vi "Read Config Settings.vi"(8 "error in (no error)":errorcluster, 10 "ConfigFile":path, 11 "Config in":refnum<class "Config.lvclass">) -> (0 "error out":errorcluster, 1 "Config Settings":T1={"Application Settings"={"Simulation"=FALSE}, "Main Settings"={"Simulation"=FALSE, "Signal scaling"=[], "ESR scaling"=[], "num readings to average"=[], "ESR alarm threshhold (%)"=[], "UseDummyVrms"=FALSE, "Dummy Vrms"=0.0, "Inverter Database File"=path "", "default Inverter (name)"=[]}, "DAQ Settings"={"Simulation"=FALSE, "Initial ErrReporting setting"=0, "Initial Measurement settings"={"Data Rate 9775"=3.0, "Data Rate 9215"=1200000.0, "Samples RMS 9215"=480000, "Samples RMS 9775"=3}, "Acquisition mode"=enum."3phase", "DemoMode"=FALSE, "RIO Device"=""}, "LogEngine Settings"={"Simulation"=FALSE, "TDMS_FolderPath"="", "CSV_FolderPath"="", "TDMS_FileName_Prefix"="", "CSV_FileName_Prefix"="", "TDMS_LogDuration(s)"=0.0, "CSV_LogDuration(s)"=0.0}} {"Main Settings"."Dummy Vrms" format="%.2g"; "DAQ Settings"."Initial ErrReporting setting" items=["DONTPRINT", "PRINTWARNINGS", "PRINTFATAL", "PRINTALL"]}, 2 "ConfigFile out":path, 3 "Config out":refnum<class "Config.lvclass">, 4 "default file created":bool)   [LabVIEW 2019, in "Config.lvclass"]
doc: "Developed by Kevin Thompson\nkevin@thompsonengineering.net\n\nCopyright 2018-2020\nThompson Engineering, LLC"
uses:
  Config.lvclass
  DataTypes/Config Settings.ctl
  Application/DataTypes/Settings--cluster.ctl
  Main/DataTypes/Settings--cluster.ctl
  Main/support/Data Algorithms/subvis/DataTypes/Gain control.ctl
  Main/support/Data Algorithms/subvis/DataTypes/ESR scaling--cluster.ctl
  DAQ_Engine/DataTypes/Settings--cluster.ctl
  Common/DataTypes/Measurement Config--cluster.ctl
  Common/DataTypes/Acquisition Mode--cluster.ctl
  Log_Engine/DataTypes/Settings--cluster.ctl
  Config.lvclass/Config.ctl
  Accessors/Set Application Settings.vi
  Accessors/Set Main Settings.vi
  Accessors/Set LogEngine Settings.vi
  <userlib>/_OpenG.lib/file/file.llb/File Exists - Scalar__ogtk.vi
  Accessors/Set DAQ Settings.vi
  Application/Application.lvclass
  DAQ_Engine/DAQ_Engine.lvclass
  Log_Engine/Log_Engine.lvclass
  Main/Main.lvclass
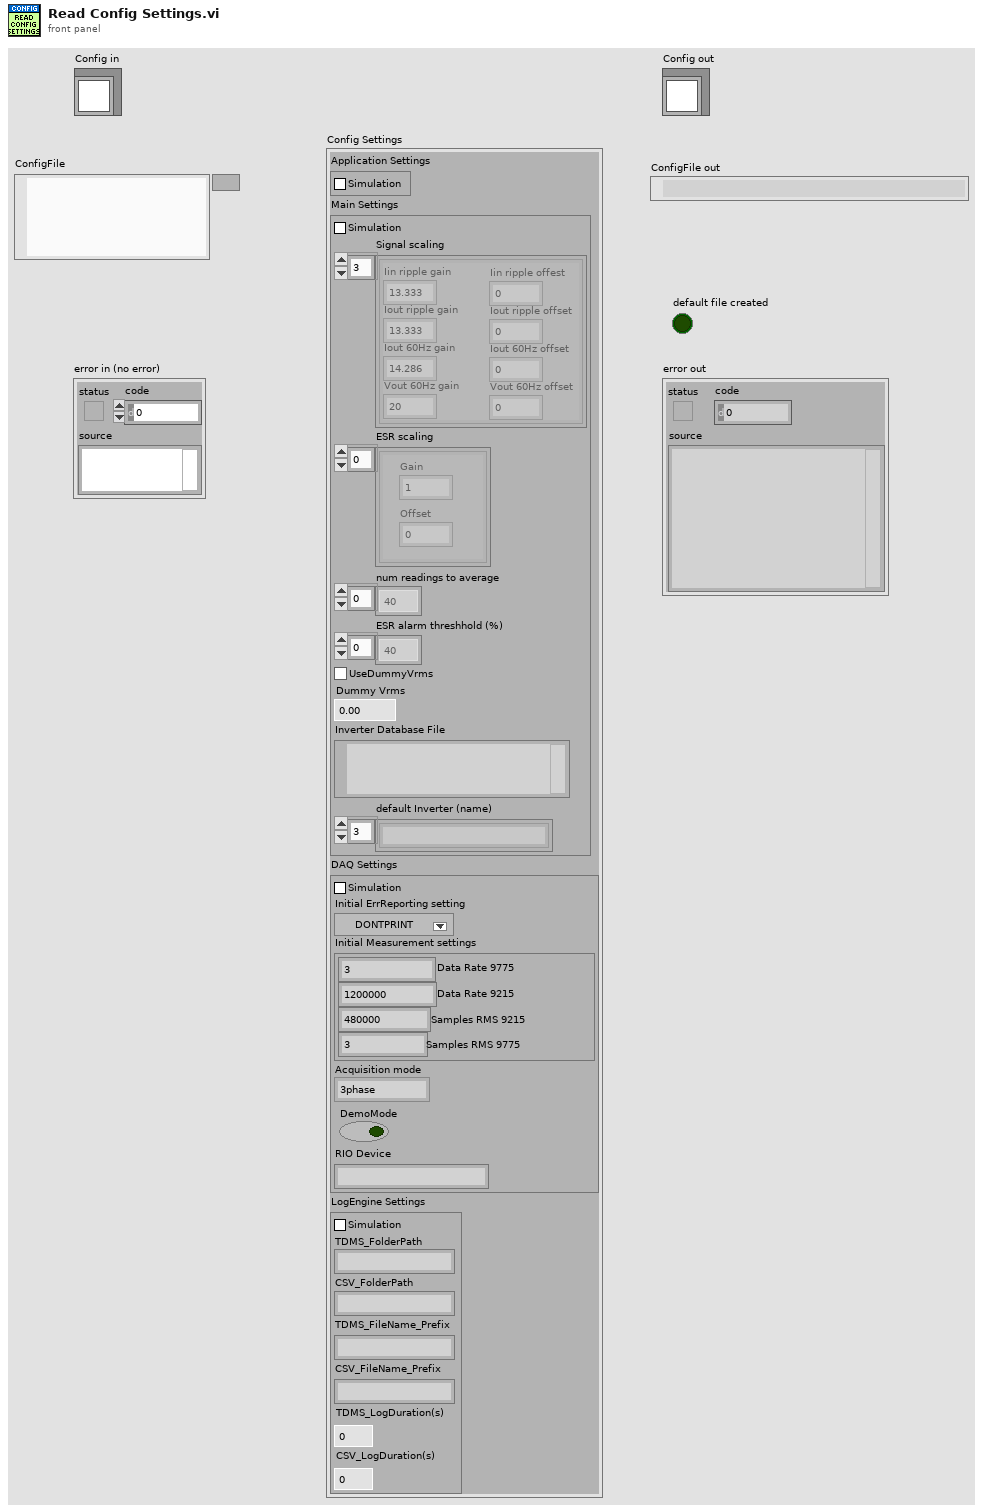
[diagram p1: front panel]
types:
  T1 = typedef "Config.lvclass/Config Settings.ctl" = cluster{"Application Settings":T2, "Main Settings":T3, "DAQ Settings":T6, "LogEngine Settings":T9}
  T2 = typedef "Application.lvclass/Settings--cluster.ctl" = cluster{"Simulation":bool}
  T3 = typedef "Main.lvclass/Settings--cluster.ctl" = cluster{"Simulation":bool, "Signal scaling":T4[], "ESR scaling":T5[], "num readings to average":i32[], "ESR alarm threshhold (%)":i32[], "UseDummyVrms":bool, "Dummy Vrms":dbl, "Inverter Database File":path, "default Inverter (name)":string[]}
  T4 = typedef "Main.lvclass/Gain control.ctl" = cluster{"Iin ripple gain":dbl, "Iout ripple gain":dbl, "Iout 60Hz gain ":dbl, "Vout 60Hz gain ":dbl, "Iin ripple offest":dbl, "Iout ripple offset":dbl, "Iout 60Hz offset":dbl, "Vout 60Hz offset":dbl}
  T5 = typedef "Main.lvclass/ESR scaling--cluster.ctl" = cluster{"Gain":dbl, "Offset":dbl}
  T6 = typedef "DAQ_Engine.lvclass/Settings--cluster.ctl" = cluster{"Simulation":bool, "Initial ErrReporting setting":i32, "Initial Measurement settings":T7, "Acquisition mode":T8, "DemoMode":bool, "RIO Device":string}
  T7 = typedef "Measurement Config--cluster.ctl" = cluster{"Data Rate 9775":dbl, "Data Rate 9215":dbl, "Samples RMS 9215":u32, "Samples RMS 9775":u32}
  T8 = typedef "Acquisition Mode--cluster.ctl" = enum16{"3phase", "Single"}
  T9 = typedef "Log_Engine.lvclass/Settings--cluster.ctl" = cluster{"Simulation":bool, "TDMS_FolderPath":string, "CSV_FolderPath":string, "TDMS_FileName_Prefix":string, "CSV_FileName_Prefix":string, "TDMS_LogDuration(s)":dbl, "CSV_LogDuration(s)":dbl}
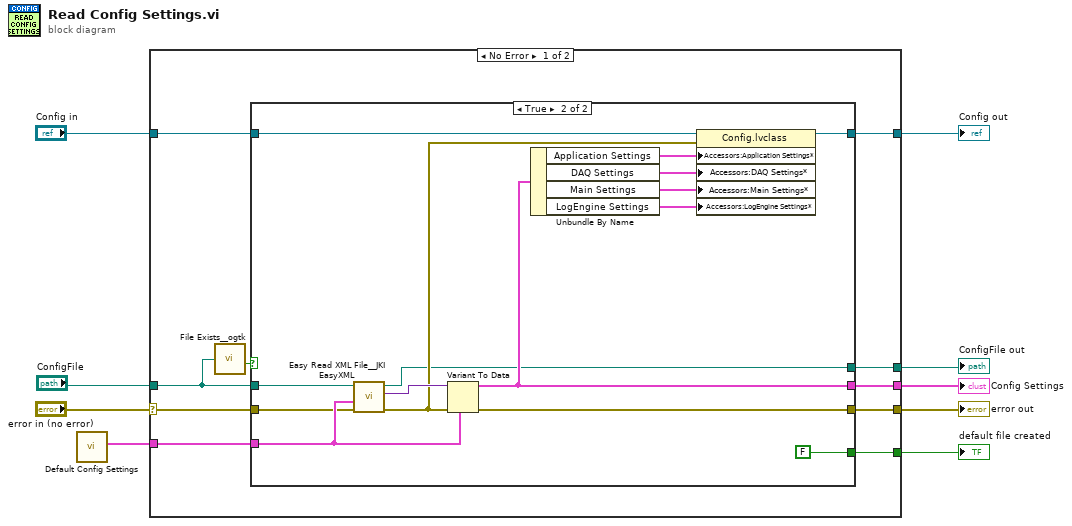
[diagram p0: block diagram]
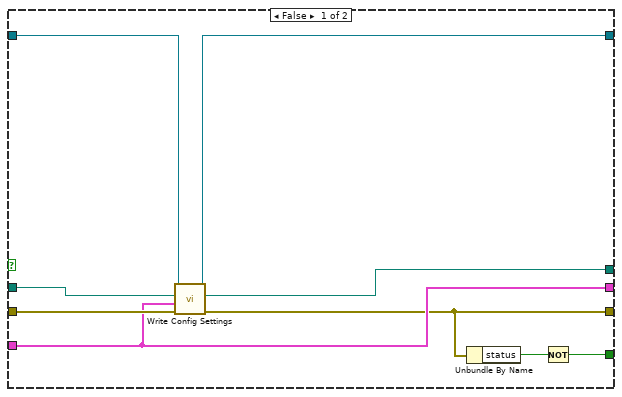
[diagram p2: hidden frame]
diagram:
  n1 = call "Default Config Settings.vi"() -> ("Config Settings"=w2:T1)  [unwired: 10 in, 1 out]
  n2 = case shown="No Error" "error in (no error)" {
    selector: "error in (no error)" -> [w17 w47]
    tunnel: [w16 w47] -> w8
    tunnel: [w13 w46] -> w6
    tunnel: "Config in" -> [w14 w46]
    tunnel: "ConfigFile" -> [w12 w44]
    tunnel: [w15 w45] -> w5
    tunnel: [w18 _] -> w3
    tunnel: w2 -> [w11 w45]
    tunnel: [w10 w44] -> w1
    frame No Error {
      n3 = call-poly <userlib>:"File Exists__ogtk.vi"("file path"=w12) -> ("exists"=w19:bool)  [unwired: 6 in, 1 out]
      n4 = case shown="True" w19 {
        tunnel: w12 -> [w27 w35]
        tunnel: [w24 w36] -> w15
        tunnel: w11 -> [w24 w34]
        tunnel: [w23 w30] -> w16
        tunnel: [w21 FALSE] -> w18
        tunnel: w17 -> [w28 w31]
        tunnel: w14 -> [w26 w38]
        tunnel: [w25 w37] -> w13
        tunnel: [w20 w29] -> w10
        frame False {
          n5 = call "Write Config Settings.vi"("error in (no error)"=w28, "Config Settings"=w24, "ConfigFile"=w27, "Config in"=w26) -> ("error out"=w23:errorcluster, "ConfigFile out"=w20:path, "Config out"=w25:refnum<class "Config.lvclass">)  [unwired: 5 in]
          n6 = Unbundle By Name(w23) -> ("status"=w22:bool)
          n7 = Not(x=w22) -> (.not. x?=w21:bool)
        }
        frame True {
          n8 = call <vilib>:"Easy Read XML File__JKI EasyXML.vi"("error in (no error)"=w31, "LabVIEW Data (Type)"=w34, "XML File Path"=w35) -> ("error out"=w32:errorcluster, "LabVIEW Data"=w33:variant, "XML File Path (duplicate)"=w29:path)  [unwired: 6 in]
          n9 = Variant To Data(error in=w32, type=w34, Variant=w33) -> (data=w36:T1, error out=w30:errorcluster)
          n10 = Unbundle By Name(w36) -> ("Application Settings"=w39:T2, "DAQ Settings"=w42:T6, "Main Settings"=w41:T3, "LogEngine Settings"=w40:T9)
          n11 = property class="Config.lvclass"(reference=w38, error in=w32, "Accessors:Application Settings*"=w39, "Accessors:DAQ Settings*"=w42, "Accessors:Main Settings*"=w41, "Accessors:LogEngine Settings*"=w40) -> (reference out=w37:refnum<class "Config.lvclass">)  [unwired: 1 out]
        }
      }
    }
    frame Error {
    }
  }
  "error out" <- w8
  "Config out" <- w6
  "Config Settings" <- w5
  "ConfigFile out" <- w1
  "default file created" <- w3
